vi "RouteGuide GetFeature.vi"(6 "contextId":T1, 7 "With Occurrence":enum16{"WithOccurrence", "WithoutOccurrence"}(ring), 8 "error in":errorcluster, 9 "timeout (ms)":i32=-1, 10 "Request Data":T3, 11 "gRPC ID":T1) -> (0 "error out":errorcluster, 2 "Response Data":T2, 3 "gRPC ID out":T1)   [LabVIEW 2019, in "route_guide_client.lvlib"]
uses:
  route_guide_client.lvlib
  <vilib>/gRPC/LabVIEW gRPC Library/Shared/grpcId.ctl
  RPC Messages/routeguide_Point.ctl
  RPC Messages/routeguide_Feature.ctl
  RPC Messages/routeguide_Feature_Flat.ctl
  RPC Messages/routeguide_Point_Flat.ctl
  14035477-4c25-4107-8ed5-d0c4ef420ce5.vi
  <vilib>/gRPC/LabVIEW gRPC Library/Shared/TranslateGrpcError.vi
  <vilib>/gRPC/LabVIEW gRPC Library/Shared/Wait On Occurence.vi
  RPC Messages/FlatToRichrouteguide_Point.vi
  <vilib>/gRPC/LabVIEW gRPC Library/Server API/Server/Get Server DLL Path.vi
  <vilib>/Utility/error.llb/Error Cluster From Error Code.vi
  <vilib>/gRPC/LabVIEW gRPC Library/grpc-lvsupport-release.lvlib
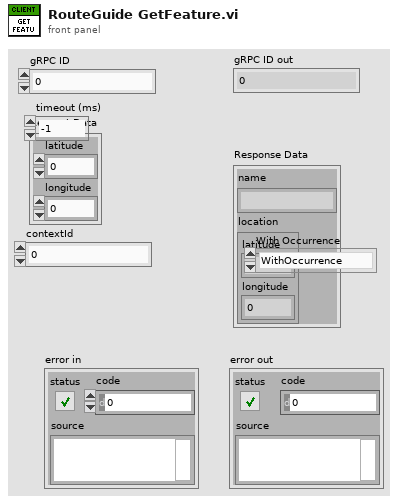
[diagram p1: front panel]
types:
  T1 = typedef "grpc-lvsupport-release.lvlib/grpcId.ctl" = u64
  T2 = typedef "route_guide_client.lvlib/routeguide_Feature.ctl" = cluster{"name":string, "location":T3}
  T3 = typedef "route_guide_client.lvlib/routeguide_Point.ctl" = cluster{"latitude":i32, "longitude":i32}
  T4 = typedef "route_guide_client.lvlib/routeguide_Feature_Flat.ctl" = cluster{"name":string, "location":T5}
  T5 = typedef "route_guide_client.lvlib/routeguide_Point_Flat.ctl" = cluster{"latitude":i32, "longitude":i32}
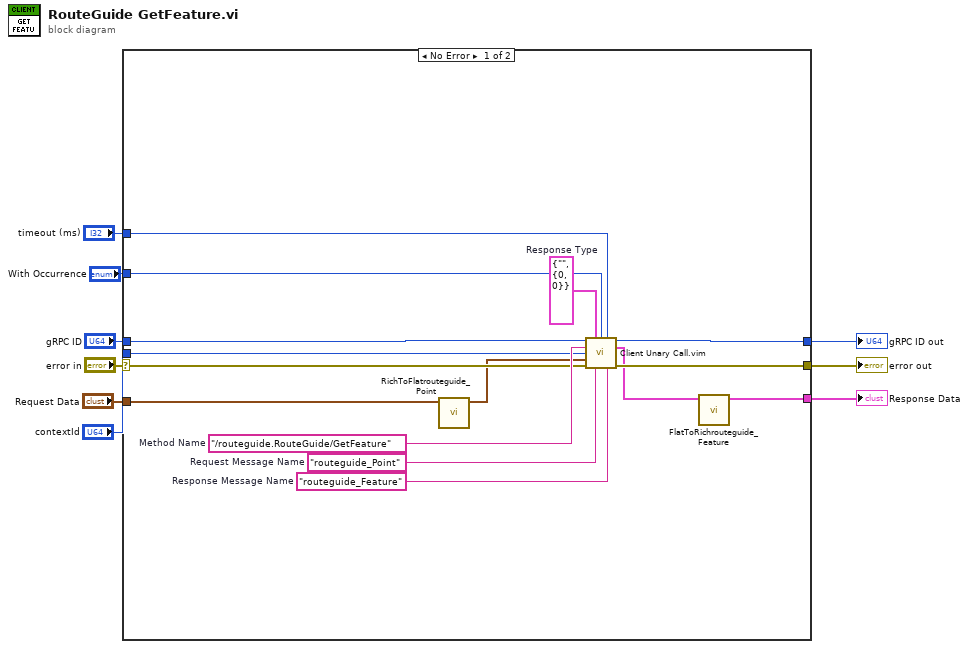
[diagram p0: block diagram]
diagram:
  n1 = case shown="No Error" "error in" {
    selector: "error in" -> [w20 w25]
    tunnel: [w19 w25] -> w8
    tunnel: "gRPC ID" -> [w18 w26]
    tunnel: [w17 w26] -> w6
    tunnel: "Request Data" -> [w14 _]
    tunnel: [w11 _] -> w4
    tunnel: "timeout (ms)" -> [w16 _]
    tunnel: "contextId" -> [w15 _]
    tunnel: "With Occurrence" -> [w10 _]
    frame No Error {
      w21 = "routeguide_Feature"  # Response Message Name
      w22 = "routeguide_Point"  # Request Message Name
      w23 = T4 {"name"="", "location"={"latitude"=0, "longitude"=0}}  # Response Type
      w24 = "/routeguide.RouteGuide/GetFeature"  # Method Name
      n2 = call "RichToFlatrouteguide_Point.vi"("InputCluster"=w14) -> ("OutputCluster"=w13:T5)  [unwired: 10 in]
      n3 = call "Client Unary Call.vim"("ClientID in"=w18, "Response Type"=w23, "Occurrence"=w10, "timeout (ms)"=w16, "Method Name"=w24, "contextId"=w15, "Request Data"=w13, "error in"=w20, "Request Message Name"=w22, "Response Message Name"=w21) -> ("ClientID out"=w17:u64, "Response Data"=w12:T4, "error out"=w19:errorcluster)  [unwired: 3 in]
      n4 = call "FlatToRichrouteguide_Feature.vi"("InputCluster"=w12) -> ("OutputCluster"=w11:T2)  [unwired: 10 in]
    }
    frame Error {
    }
  }
  "error out" <- w8
  "gRPC ID out" <- w6
  "Response Data" <- w4
